vi "ZeroMQ_PUBGS.vi"() -> ()   [LabVIEW 2018]
uses:
  <vilib>/addons/zeromq/socket_type.ctl
  <vilib>/addons/zeromq/zeromq.lvlib
  <vilib>/addons/zeromq/zmq_context.lvclass
  <vilib>/addons/zeromq/zmq_socket.lvclass
panel:
  out "timed out?":bool
  out "pub":string
  out "error out 2":errorcluster
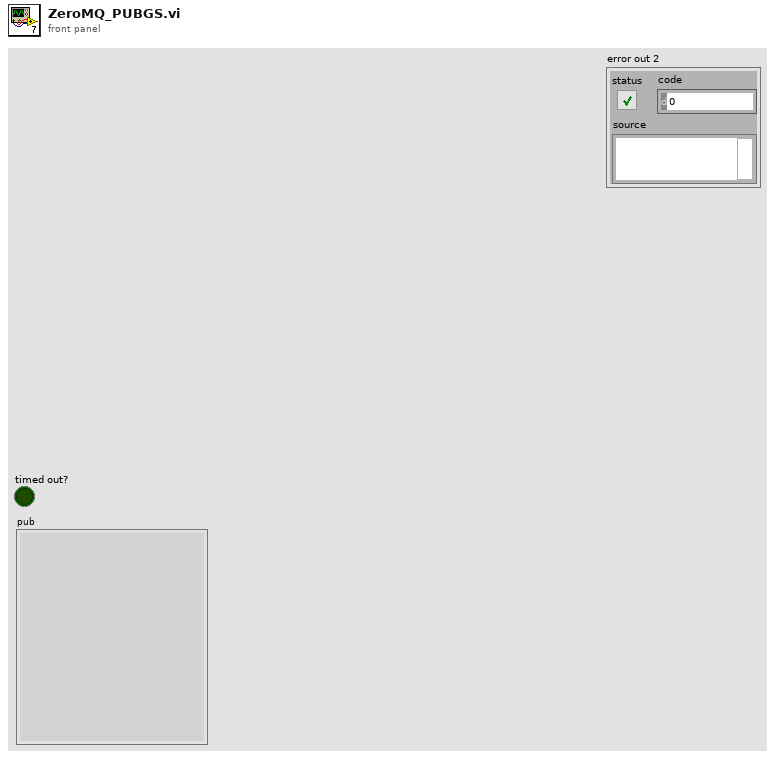
[diagram p1: front panel]
types:
  T1 = typedef "zeromq.lvlib/socket_type.ctl" = enum8{"ZMQ_PAIR", "ZMQ_PUB", "ZMQ_SUB", "ZMQ_REQ", "ZMQ_REP", "ZMQ_DEALER", "ZMQ_ROUTER", "ZMQ_PULL", "ZMQ_PUSH", "ZMQ_XPUB", "ZMQ_XSUB", "ZMQ_STREAM", "ZMQ_SERVER", "ZMQ_CLIENT", "ZMQ_RADIO", "ZMQ_DISH", "ZMQ_GATHER", "ZMQ_SCATTER", "ZMQ_DGRAM"}
  T2 = cluster{"ID":u32, "Address":string, "Service Name 1":string, "Service Name 2":string, "queue TX":refnum<queue>, "queue RX":refnum<queue>, "Port 1":u32, "Port 2":u32}
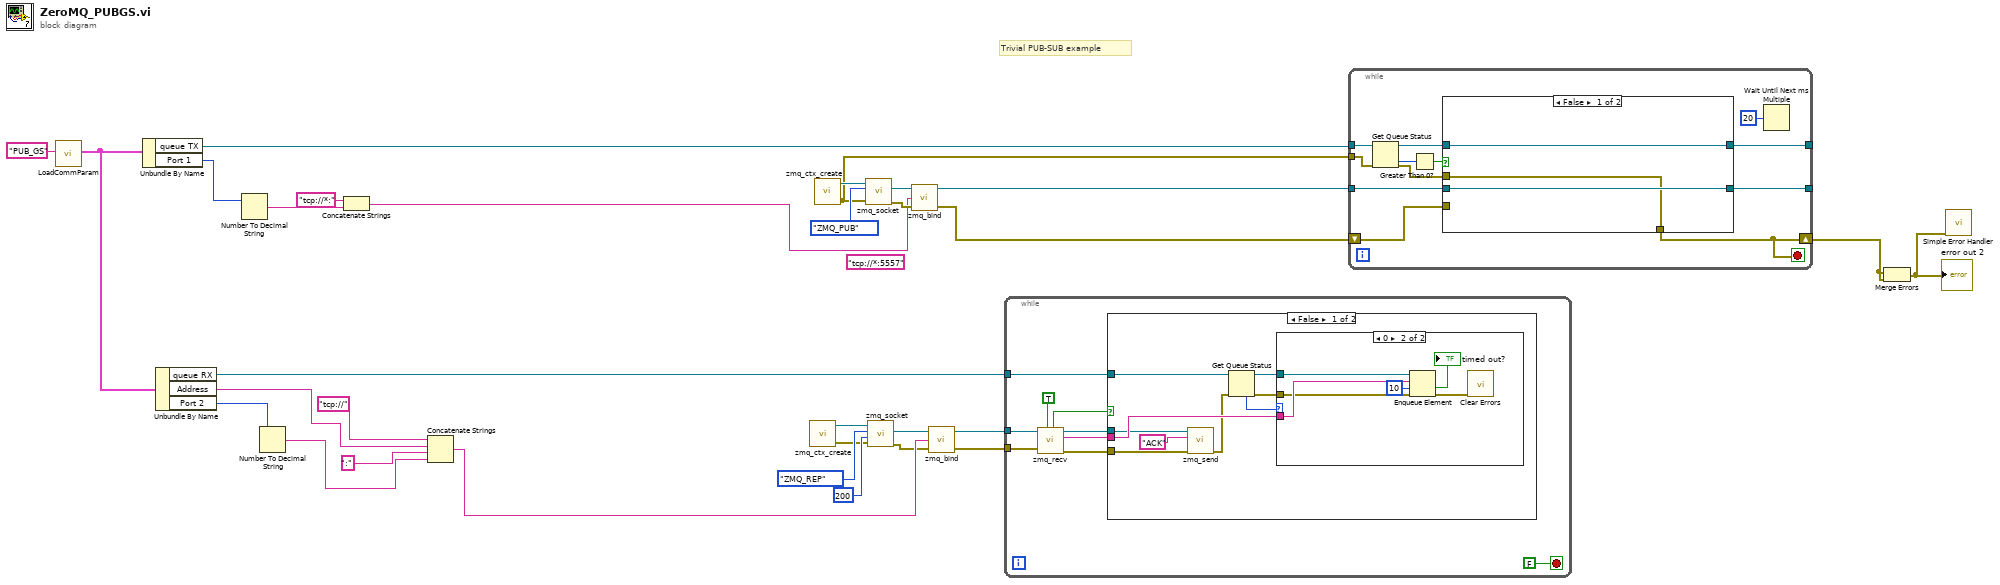
[diagram p0: block diagram]
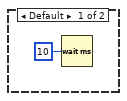
[diagram p2: hidden frame]
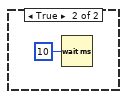
[diagram p3: hidden frame]
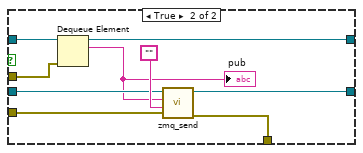
[diagram p4: hidden frame]
diagram:
  (unwired) "tcp://*:5557" ("endpoint")
  # "Trivial PUB-SUB example"
  n1 = call "LoadCommParam.vi"("section name"="PUB_GS") -> ("output cluster"=w11:T2)  [unwired: 10 in]
  n2 = Unbundle By Name(w11) -> ("queue TX"=w20:refnum<queue>, "Port 1"=w24:u32)
  n3 = Unbundle By Name(w11) -> ("queue RX"=w10:refnum<queue>, "Address"=w8:string, "Port 2"=w5:u32)
  n4 = Number To Decimal String(number=w24) -> (decimal integer string=w23:string)  [unwired: 1 in]
  n5 = Number To Decimal String(number=w5) -> (decimal integer string=w6:string)  [unwired: 1 in]
  n6 = Concatenate Strings("tcp://*:" ("string"), w23) -> (w19:string)
  n7 = Concatenate Strings("tcp://" ("string"), w8, ":" ("string"), w6) -> (w4:string)
  n8 = call <vilib>:"zmq_ctx_create.vi"() -> ("error out"=w3:errorcluster, "context out"=w14:refnum<class "zmq_context.lvclass">)  [unwired: 4 in]
  n9 = call <vilib>:"zmq_ctx_create.vi"() -> ("error out"=w21:errorcluster, "context out"=w31:refnum<class "zmq_context.lvclass">)  [unwired: 4 in]
  n10 = call <vilib>:"zmq_socket.vi"("error in"=w21, "socket type"=socket_type."ZMQ_PUB", "context in"=w31) -> ("error out"=w28:errorcluster, "socket out"=w29:refnum<class "zmq_socket.lvclass">)  [unwired: 2 in, 1 out]
  n11 = call <vilib>:"zmq_socket.vi"("error in"=w3, "linger (ms)"=200, "socket type"=socket_type."ZMQ_REP", "context in"=w14) -> ("error out"=w2:errorcluster, "socket out"=w13:refnum<class "zmq_socket.lvclass">)  [unwired: 1 in, 1 out]
  n12 = call <vilib>:"zmq_bind.vi"("error in"=w28, "endpoint"=w19, "socket in"=w29) -> ("error out"=w26:errorcluster, "socket out"=w27:refnum<class "zmq_socket.lvclass">)  [unwired: 1 in]
  n13 = call <vilib>:"zmq_bind.vi"("error in"=w2, "endpoint"=w4, "socket in"=w13) -> ("error out"=w1:errorcluster, "socket out"=w12:refnum<class "zmq_socket.lvclass">)  [unwired: 1 in]
  n14 = while {
    tunnel: w12 -> [w36]
    tunnel: w10 -> [w34]
    tunnel: w1 -> [w33]
    stop <- FALSE stop-if-true
    n15 = call <vilib>:"zmq_recv.vi"("no block? (F)"=TRUE, "error in"=w33, "socket in"=w36) -> ("error out"=w32:errorcluster, "data"=w38:string, "socket out"=w35:refnum<class "zmq_socket.lvclass">, "timeout?"=w39:bool)  [unwired: 2 in, 1 out]
    n16 = case shown="False" w39 {
      tunnel: w38 -> [w48 _]
      tunnel: w35 -> [w47 _]
      tunnel: w34 -> [w45 _]
      tunnel: w32 -> [w46 _]
      frame False {
        n17 = call <vilib>:"zmq_send.vi"("error in"=w46, "data"="ACK", "socket in"=w47) -> ("error out"=w44:errorcluster)  [unwired: 4 in, 1 out]
        n18 = Get Queue Status(queue=w45, error in (no error)=w44) -> (queue out=w42:refnum<queue>, error out=w43:errorcluster, # elements in queue=w41:i32)  [unwired: 1 in, 5 out]
        n19 = case shown="0" w41 {
          tunnel: w48 -> [_ w56]
          tunnel: w43 -> [_ w52]
          tunnel: w42 -> [_ w51]
          frame Default {
            n20 = Wait (ms)(milliseconds to wait=u32 10) -> ()  [unwired: 1 out]
          }
          frame 0 {
            n21 = Enqueue Element(queue=w51, element=w56, timeout in ms (-1)=10, error in (no error)=w52) -> (timed out?=→"timed out?":bool, error out=w55:errorcluster)  [unwired: 1 out]
            n22 = call <vilib>:"Clear Errors.vi"("error in (no error)"=w55) -> ()  [unwired: 5 in, 2 out]
          }
        }
      }
      frame True {
        n23 = Wait (ms)(milliseconds to wait=u32 10) -> ()  [unwired: 1 out]
      }
    }
  }
  n24 = while {
    tunnel: w27 -> [w65]
    tunnel: w20 -> [w69]
    tunnel: [w63] -> _
    tunnel: [w64] -> _
    tunnel: w21 -> [w62]
    shift-right: [w59] -> w17
    shift-left: w26 -> [w60]
    stop <- w59 stop-if-true
    n25 = Get Queue Status(queue=w69, error in (no error)=w62) -> (queue out=w68:refnum<queue>, error out=w61:errorcluster, # elements in queue=w67:i32)  [unwired: 1 in, 5 out]
    n26 = Greater Than 0?(x=w67) -> (x > 0?=w66:bool)
    n27 = case shown="False" w66 {
      tunnel: w68 -> [w71 w81]
      tunnel: w65 -> [w72 w79]
      tunnel: [w72 w77] -> w64
      tunnel: [w71 w78] -> w63
      tunnel: w61 -> [w70 w76]
      tunnel: [w70 w74] -> w59
      tunnel: w60 -> [_ w75]
      frame False {
      }
      frame True {
        n28 = Dequeue Element(queue=w81, error in (no error)=w76) -> (queue out=w78:refnum<queue>, element=w73:string)  [unwired: 1 in, 2 out]
        "pub" <- w73
        n29 = call <vilib>:"zmq_send.vi"("error in"=w75, "group"="", "data"=w73, "socket in"=w79) -> ("error out"=w74:errorcluster, "socket out"=w77:refnum<class "zmq_socket.lvclass">)  [unwired: 3 in]
      }
    }
    n30 = Wait Until Next ms Multiple(millisecond multiple=u32 20) -> ()  [unwired: 1 out]
  }
  n31 = Merge Errors(w17, w17) -> (w18:errorcluster)
  "error out 2" <- w18
  n32 = call <vilib>:"Simple Error Handler.vi"("error in (no error)"=w18) -> ()  [unwired: 4 in, 5 out]
